vi "add.vi"(8 "error in (no error)":errorcluster, 10 "Shape":refnum<class "Shape.lvclass">, 11 "CompoundShape in":refnum<class "CompoundShape.lvclass">) -> (0 "error out":errorcluster, 3 "CompoundShape out":refnum<class "CompoundShape.lvclass">)   [LabVIEW 2017, in "CompoundShape.lvclass"]
uses:
  CompoundShape.lvclass
  Shape Class/Shape.lvclass
  CompoundShape.lvclass/CompoundShape.ctl
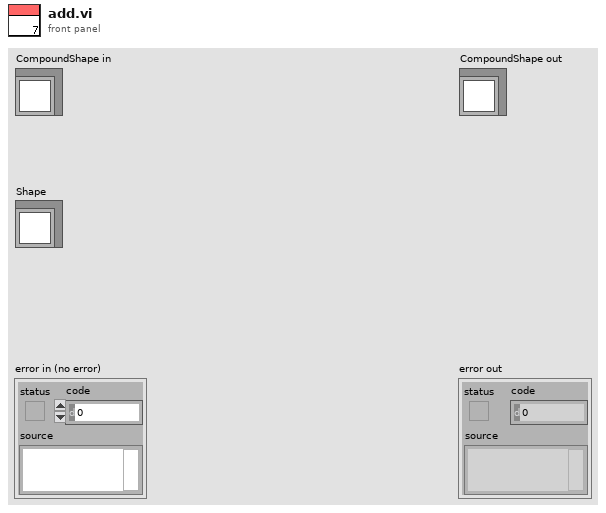
[diagram p1: front panel]
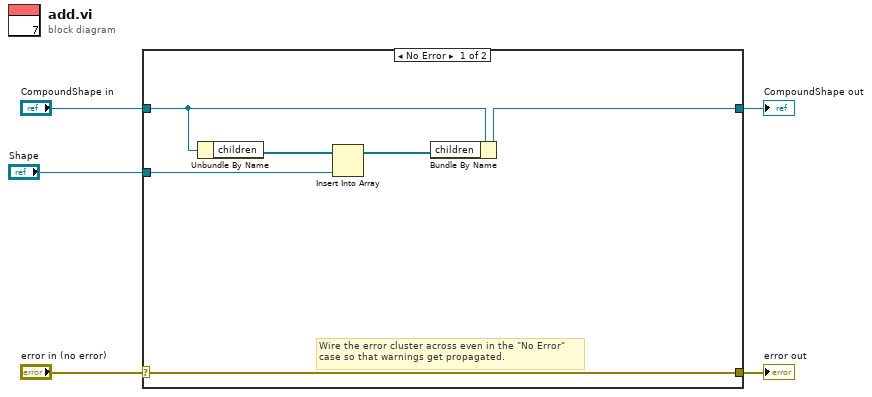
[diagram p0: block diagram]
diagram:
  n1 = case shown="No Error" "error in (no error)" {
    selector: "error in (no error)" -> [w11 w13]
    tunnel: [w11 w13] -> w4
    tunnel: [w9 w12] -> w2
    tunnel: "CompoundShape in" -> [w10 w12]
    tunnel: "Shape" -> [w6 _]
    frame No Error {
      # "Wire the error cluster across even in the \"No Error\"\ncase so that warnings get propagated."
      n2 = Unbundle By Name(w10) -> ("children"=w8:refnum<class "Shape.lvclass">[])
      n3 = Insert Into Array "Insert Into Array"(array=w8, new element=w6) -> (w7:refnum<class "Shape.lvclass">[])  [unwired: 1 in]
      n4 = Bundle By Name(cluster=w10, "children"=w7) -> (w9:refnum<class "CompoundShape.lvclass">)
    }
    frame Error {
    }
  }
  "error out" <- w4
  "CompoundShape out" <- w2
